vi "simple control module.vi"(8 "dt":dbl, 9 "results in":T2, 10 "parameters in":T2, 11 "sample control module":T1={"setpoint index (dbl)"=0, "proc var index (dbl)"=0, "output index (dbl)"=0, "output range"={"output high"=100.0, "output low"=-100.0}, "Kp"=0.0, "Ki"=0.0, "Kd"=0.0, "error int"=0.0, "last error"=0.0} {"output range"."output low" format="%.2f"; "output range"."output high" format="%.2f"}) -> (1 "results out":T2, 2 "parameters out":T2, 3 "sample control module out":T1={"setpoint index (dbl)"=0, "proc var index (dbl)"=0, "output index (dbl)"=0, "output range"={"output high"=100.0, "output low"=-100.0}, "Kp"=0.0, "Ki"=0.0, "Kd"=0.0, "error int"=0.0, "last error"=0.0} {"output range"."output low" format="%.2f"; "output range"."output high" format="%.2f"})   [LabVIEW 2013, in "configuration tests.lvlib" / "TEST RUNTIME.lvclass"]
uses:
  TEST RUNTIME.lvclass
  <vilib>/NI/Tag Bus/table/data table.ctl
  control module.ctl
  <vilib>/NI/Tag Bus/table/data polymorphs/read one/read Double.vi
  <vilib>/NI/Tag Bus/table/data polymorphs/write one/write Double.vi
  <vilib>/NI/Tag Bus/table/data table.lvlib
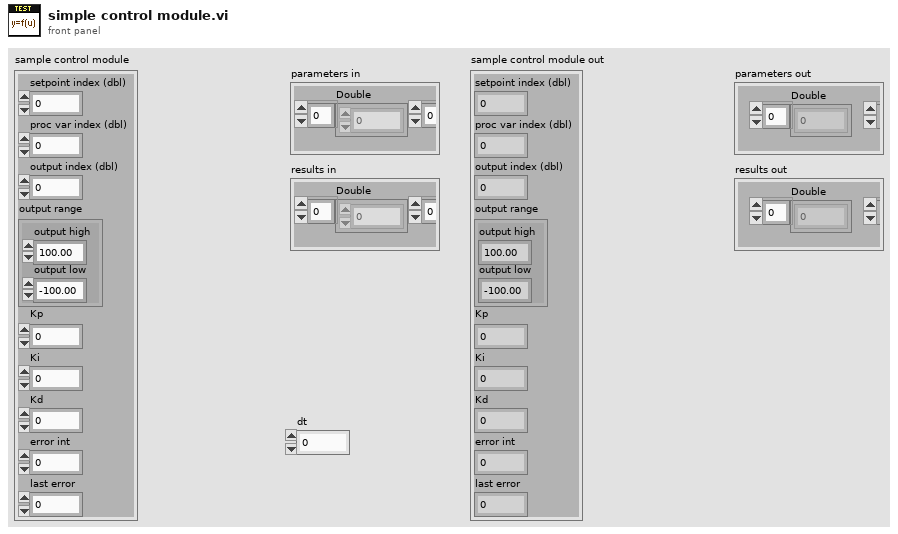
[diagram p1: front panel]
types:
  T1 = typedef "configuration tests.lvlib/TEST RUNTIME.lvclass/control module.ctl" = cluster{"setpoint index (dbl)":i32, "proc var index (dbl)":i32, "output index (dbl)":i32, "output range":cluster{"output high":dbl, "output low":dbl}, "Kp":dbl, "Ki":dbl, "Kd":dbl, "error int":dbl, "last error":dbl}
  T2 = typedef "tag bus.lvlib/data table.lvlib/data table.ctl" = cluster{"Double":dbl[], "Single":sgl[], "I64":i64[], "I32":i32[], "I16":i16[], "I8":i8[], "U64":u64[], "U32":u32[], "U16":u16[], "U8":u8[], "Boolean":bool[], "String":string[], "Array of Double":cluster{"DBL Array":dbl[]}[], "Array of Single":cluster{"SGL Array":sgl[]}[], "Array of I64":cluster{"I64 Array":i64[]}[], "Array of I32":cluster{"I32 Array":i32[]}[], "Array of I16":cluster{"I16 Array":i16[]}[], "Array of I8":cluster{"I8 Array":i8[]}[], "Array of U64":cluster{"U64 Array":u64[]}[], "Array of U32":cluster{"U32 Array":u32[]}[], "Array of U16":cluster{"U16 Array":u16[]}[], "Array of U8":cluster{"U8 Array":u8[]}[], "Array of Boolean":cluster{"Boolean Array":bool[]}[], "Array of String":cluster{"String Array":string[]}[]}
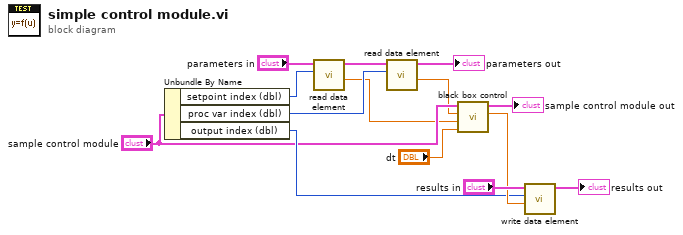
[diagram p0: block diagram]
diagram:
  n1 = Unbundle By Name("sample control module") -> ("setpoint index (dbl)"=w7:i32, "proc var index (dbl)"=w6:i32, "output index (dbl)"=w5:i32)
  n2 = call-poly <vilib>:"read data element.vi"("index"=w7, "data table in"="parameters in") -> ("value"=w1:dbl, "data table out"=w10:T2)  [unwired: 8 in]
  n3 = call-poly <vilib>:"read data element.vi"("index"=w6, "data table in"=w10) -> ("value"=w2:dbl, "data table out"=→"parameters out":T2)  [unwired: 8 in]
  n4 = call "black box control.vi"("dt"="dt", "setpoint"=w1, "process variable"=w2, "sample control module in"="sample control module") -> ("output high"=w8:dbl, "sample control module out"=→"sample control module out":T1)  [unwired: 6 in]
  n5 = call-poly <vilib>:"write data element.vi"("value"=w8, "index"=w5, "data table in"="results in") -> ("data table out"=→"results out":T2)  [unwired: 8 in]
